vi "battaglia.vi"(4 "d3 difesa":dbl, 6 "d2 difesa":dbl, 8 "d1 difesa":dbl, 9 "d3 attacco":dbl, 10 "d2 attacco":dbl, 11 "d1 attacco":dbl) -> (3 "risultati battaglia":bool[](array[boolean]))   [LabVIEW 2013]
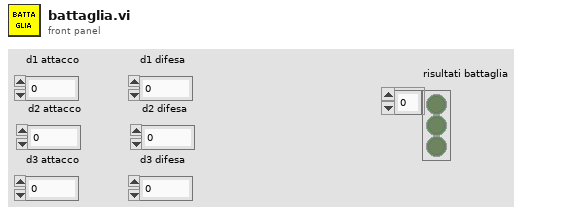
[diagram p1: front panel]
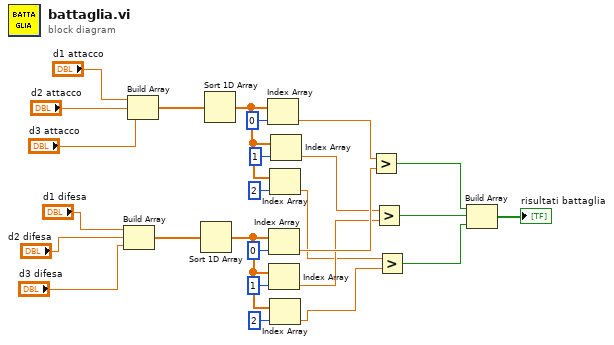
[diagram p0: block diagram]
diagram:
  n1 = Build Array("d1 difesa", "d2 difesa", "d3 difesa") -> (w26:dbl[])
  n2 = Build Array("d1 attacco", "d2 attacco", "d3 attacco") -> (w25:dbl[])
  n3 = Sort 1D Array(array=w26) -> (sorted array=w23:dbl[])
  n4 = Sort 1D Array(array=w25) -> (sorted array=w24:dbl[])
  n5 = Index Array(array=w24, index=0) -> (element=w16:dbl)
  n6 = Index Array(array=w23, index=0) -> (element=w15:dbl)
  n7 = Index Array(array=w23, index=1) -> (element=w13:dbl)
  n8 = Index Array(array=w24, index=2) -> (element=w12:dbl)
  n9 = Index Array(array=w23, index=2) -> (element=w11:dbl)
  n10 = Index Array(array=w24, index=1) -> (element=w14:dbl)
  n11 = Greater?(x=w16, y=w15) -> (0:w4:bool)
  n12 = Greater?(x=w14, y=w13) -> (0:w3:bool)
  n13 = Greater?(x=w12, y=w11) -> (0:w2:bool)
  n14 = Build Array(w4, w3, w2) -> (→"risultati battaglia":bool[])
